vi "elapsed.vi"(4 "INIT?":bool) -> (2 "min":dbl, 3 "sec":dbl)   [LabVIEW 2014]
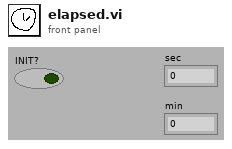
[diagram p1: front panel]
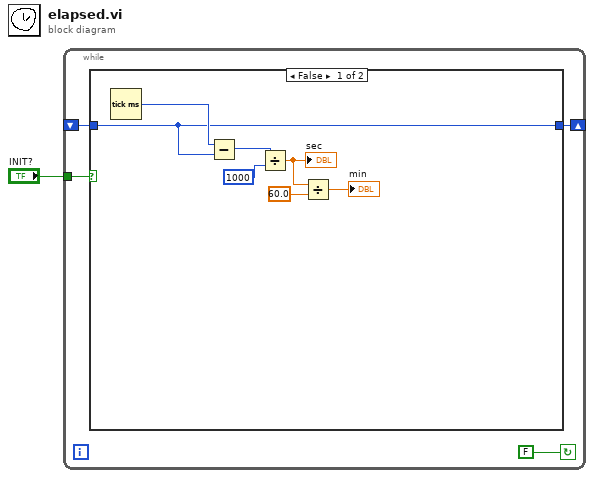
[diagram p0: block diagram]
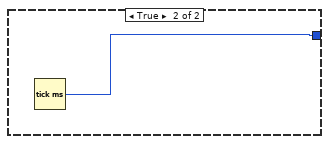
[diagram p2: hidden frame]
diagram:
  n1 = while {
    tunnel: "INIT?" -> [w5]
    shift-right: [w4] -> _
    shift-left: _ -> [w3]
    stop <- FALSE continue-if-true
    n2 = case shown="False" w5 {
      tunnel: [w9 w13] -> w4
      tunnel: w3 -> [w9 _]
      frame False {
        n3 = Tick Count (ms)() -> (millisecond timer value=w10:u32)
        n4 = Subtract(x=w10, y=w9) -> (x-y=w12:u32)
        n5 = Divide(x=w12, y=u32 1000) -> (x/y=w8:dbl)
        "sec" <- w8
        n6 = Divide(x=w8, y=60.0) -> (x/y=→"min":dbl)
      }
      frame True {
        n7 = Tick Count (ms)() -> (millisecond timer value=w13:u32)
      }
    }
  }
